vi "Table_ToolConfiguration.vi"(7 "Action":T1, 8 "error in":errorcluster, 10 "Custom Data":T2={"Channel Selection"=[], "Widths"=[], "Sort Info"={"Order"=enum."ascending", "Column"=0}, "Listbox Settings"={"Font"=13, "Bold"=FALSE, "Poll Rate"=200, "Enable Limits"=FALSE, "Path"=path ""}}, 11 "datalog path (use dialog)":path) -> (0 "error out":errorcluster, 2 "Custom Data Out":T2, 3 "path out":path)   [LabVIEW 2012, in "TableSupportLib.lvlib"]
uses:
  TableSupportLib.lvlib
  Table_StateInformation.ctl
  Table_ChannelInfoCluster.ctl
  Table_SortArraySettings.ctl
  Table_ListboxSettings.ctl
  Table_ToolConfiguration_Action.ctl
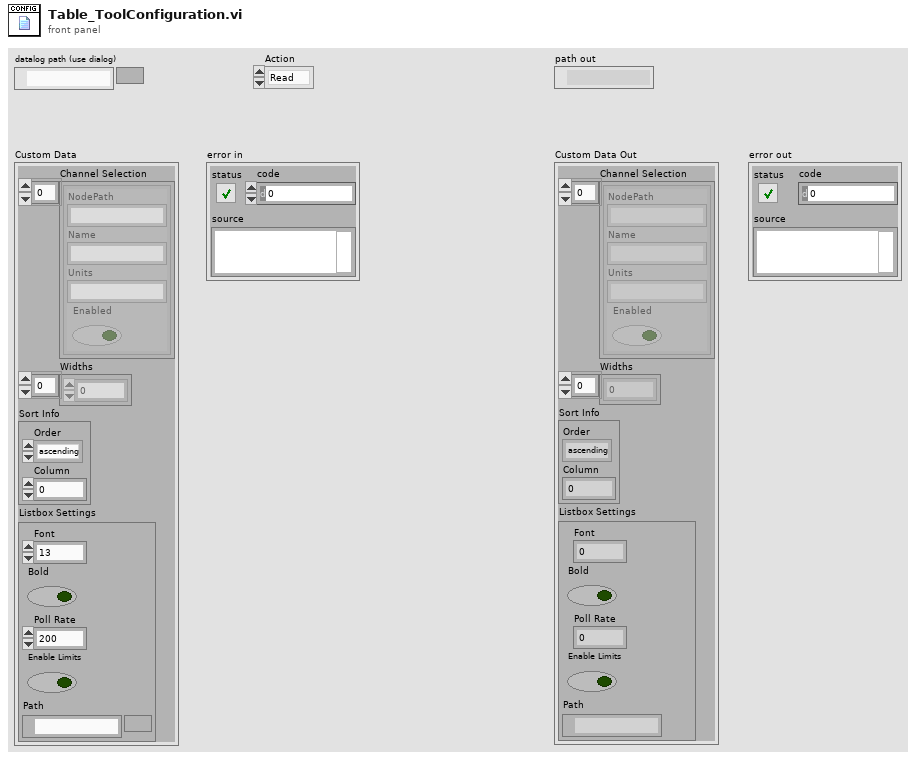
[diagram p1: front panel]
types:
  T1 = typedef "TableSupportLib.lvlib/Table_ToolConfiguration_Action.ctl" = enum16{"Read", "Write"}
  T2 = typedef "TableSupportLib.lvlib/Table_StateInformation.ctl" = cluster{"Channel Selection":T3[], "Widths":dbl[], "Sort Info":T4, "Listbox Settings":T5}
  T3 = typedef "TableSupportLib.lvlib/Table_ChannelInfoCluster.ctl" = cluster{"NodePath":string, "Name":string, "Units":string, "Enabled":bool}
  T4 = typedef "TableSupportLib.lvlib/Table_SortArraySettings.ctl" = cluster{"Order":enum16{"ascending", "descending"}, "Column":i32}
  T5 = typedef "TableSupportLib.lvlib/Table_ListboxSettings.ctl" = cluster{"Font":u32, "Bold":bool, "Poll Rate":u32, "Enable Limits":bool, "Path":path}
  T6 = enum16{"open", "replace", "create", "open or create", "replace or create", "replace or create with confirmation"}
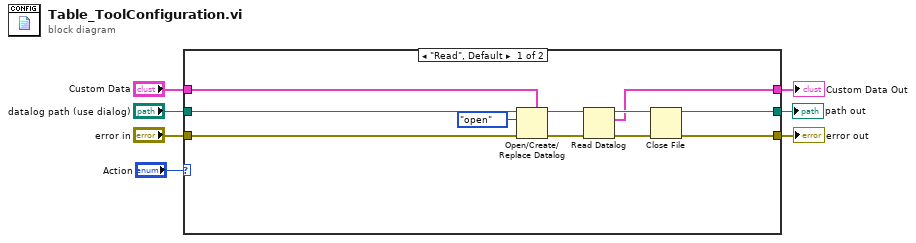
[diagram p0: block diagram]
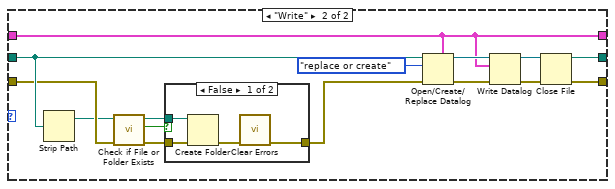
[diagram p2: hidden frame]
diagram:
  n1 = case shown="\"Read\", Default" "Action" {
    tunnel: "Custom Data" -> [w14 w29]
    tunnel: [w12 w29] -> w5
    tunnel: "datalog path (use dialog)" -> [w11 w26]
    tunnel: [w10 w27] -> w4
    tunnel: "error in" -> [w9 w25]
    tunnel: [w8 w19] -> w1
    frame "Read", Default {
      n2 = Open/Create/Replace Datalog(5:w14, 8:w9, 10:T6."open" ("operation (0:open)"), 11:w11) -> (0:w18:errorcluster, 3:w17:refnum<k1>)  [unwired: 2 in, 1 out]
      n3 = Read Datalog(4:w18, 7:w17) -> (0:w16:errorcluster, 2:w12:T2, 3:w15:refnum<k1>)  [unwired: 1 in]
      n4 = Close File(refnum=w15, error in=w16) -> (path=w8:path, error out=w10:errorcluster)
    }
    frame "Write" {
      n5 = Strip Path(path=w26) -> (stripped path=w24:path)  [unwired: 1 out]
      n6 = call <vilib>:"Check if File or Folder Exists.vi"("error in (no error)"=w25, "path"=w24) -> ("error out"=w23:errorcluster, "file or folder exists?"=w20:bool, "dup path"=w22:path)  [unwired: 7 in]
      n7 = case shown="False" w20 {
        tunnel: w23 -> [w37 w38]
        tunnel: w22 -> [w36 _]
        tunnel: [w34 w38] -> w21
        frame False {
          n8 = Create Folder(path (use dialog)=w36, error in=w37) -> (error out=w35:errorcluster)  [unwired: 1 in, 2 out]
          n9 = call <vilib>:"Clear Errors.vi"("error in (no error)"=w35) -> ("error out"=w34:errorcluster)  [unwired: 6 in]
        }
        frame True {
        }
      }
      n10 = Open/Create/Replace Datalog(5:w29, 8:w21, 10:T6."replace or create" ("operation (0:open)"), 11:w26) -> (0:w33:errorcluster, 3:w32:refnum<k1>)  [unwired: 2 in, 1 out]
      n11 = Write Datalog(4:w33, 6:w29, 7:w32) -> (0:w30:errorcluster, 3:w28:refnum<k1>)
      n12 = Close File(refnum=w28, error in=w30) -> (path=w19:path, error out=w27:errorcluster)
    }
  }
  "Custom Data Out" <- w5
  "error out" <- w4
  "path out" <- w1
